vi "Timer.vi"() -> ()   [LabVIEW 2021]
uses:
  <vilib>/MakerHub/LINX/Public/Peripherals/Digital/Digital Read 1 Chan.vi
  <vilib>/MakerHub/LINX/Public/Peripherals/Digital/Digital Read N Chans.vi
  <vilib>/MakerHub/LINX/Public/Peripherals/Digital/Digital Write N Chans.vi
  <vilib>/MakerHub/LINX/Private/Local IO/LinxDigitalRead.vi
  <vilib>/MakerHub/LINX/Public/Utilities/Check Channel.vi
  <vilib>/MakerHub/LINX/Private/Local IO/LinxDigitalWrite.vi
  <vilib>/MakerHub/LINX/Public/Utilities/Open Serial.vi
  <vilib>/MakerHub/LINX/Private/Utilties/Generate Error.vi
  <vilib>/MakerHub/LINX/Public/Peripherals/Digital/Digital Write 1 Chan.vi
  <vilib>/MakerHub/LINX/LMH-LINX.lvlib
panel:
  in  "Physical Alarm Channel":u8
  out "Clock Pulse":bool
  in  "Clock Probe Channel":u8
  in  "Serial Port":refnum<visa-resource-name>="N/A"
  out "Alarm":bool
  in  "?":bool
  in  "Seconds":dbl
  in  "Minutes":dbl
  out "timer output\ntimer output":string
  in  "?":bool
  # "LINX Settings"
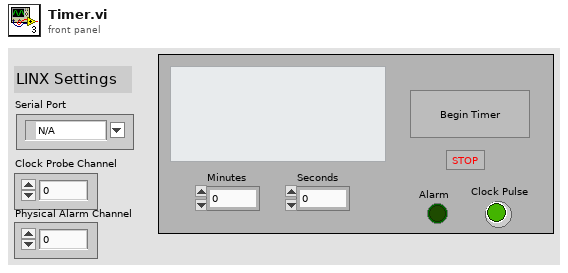
[diagram p1: front panel]
types:
  T1 = enum16{"Set Timer", "Show Running Timer", "Timer Complete", "Done"}
  T2 = typedef "LMH-LINX.lvlib/LINX Ref.ctl" = cluster{"IO":T3, "Interface":T4, "LINX Device Config":T5}
  T3 = typedef "LMH-LINX.lvlib/Platform.ctl" = enum16{"Remote", "Local"}
  T4 = typedef "LMH-LINX.lvlib/Interface.ctl" = enum16{"Serial", "TCP"}
  T5 = typedef "LMH-LINX.lvlib/Device.lvlib/LINX Device Config.ctl" = cluster{"Interface":T4, "COM Port":refnum<visa-resource-name>, "TCP Configuration":T6, "Device Family":u8, "Device ID":u8, "Device Name":string, "TCP Ref":refnum<k5>, "Channels":T7}
  T6 = typedef "LMH-LINX.lvlib/Device.lvlib/TCP Config.ctl" = cluster{"IP Address":string, "Port":u16}
  T7 = typedef "LMH-LINX.lvlib/Channels.ctl" = cluster{"DI":u8[], "DO":u8[], "AI":u8[], "AO":u8[], "PWM":u8[], "QE":u8[], "UART":u8[], "I2C 2":u8[], "SPI":u8[], "CAN":u8[], "Servo":u8[], "AI Ref (V)":dbl, "AI Resolution (Bits)":u8, "AO Ref (V)":dbl, "AO Resolution (Bits)":u8}
  T8 = enum16{"Set Timer", "Show Running Timer", "Timer Complete"}
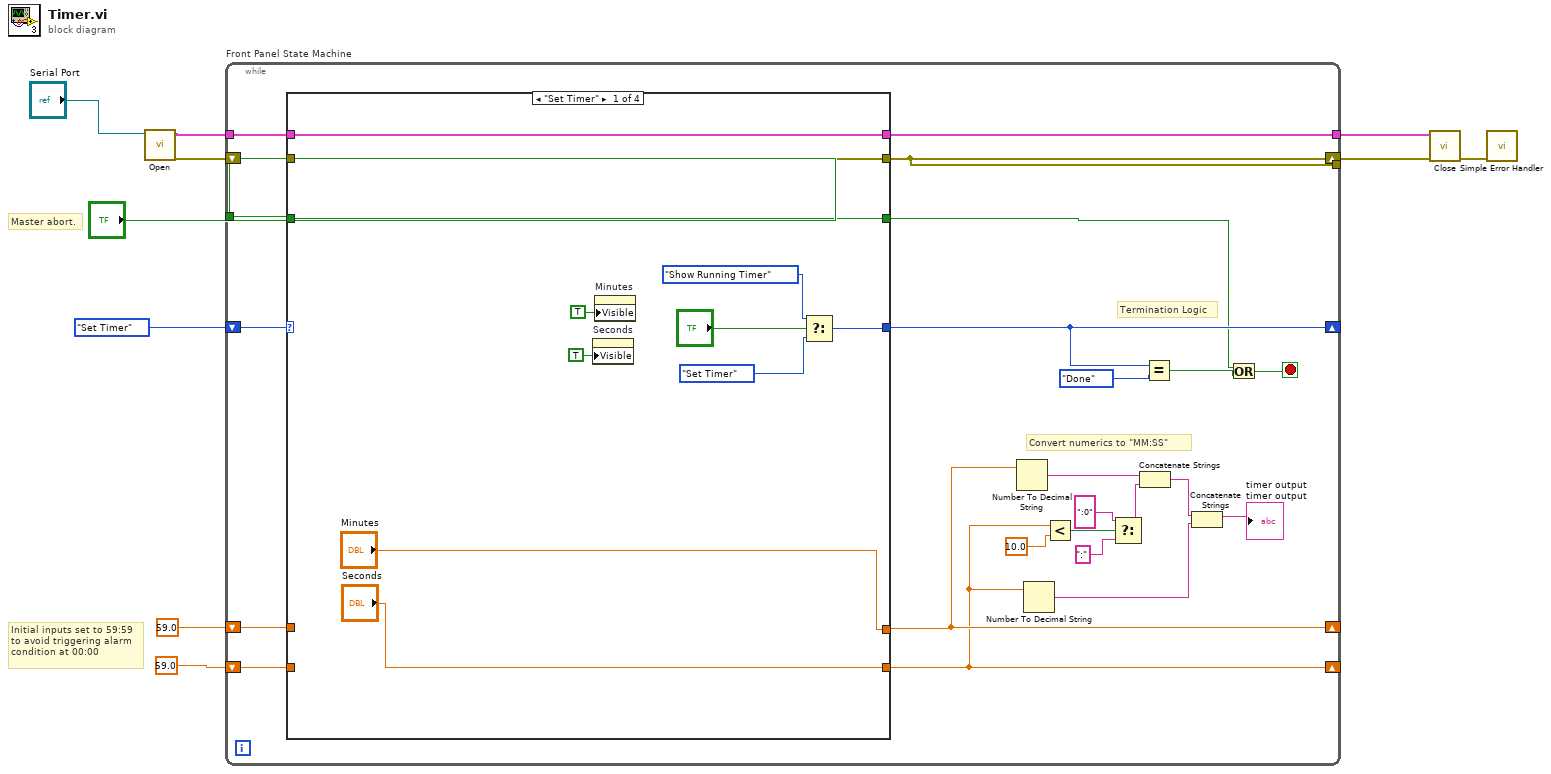
[diagram p0: block diagram]
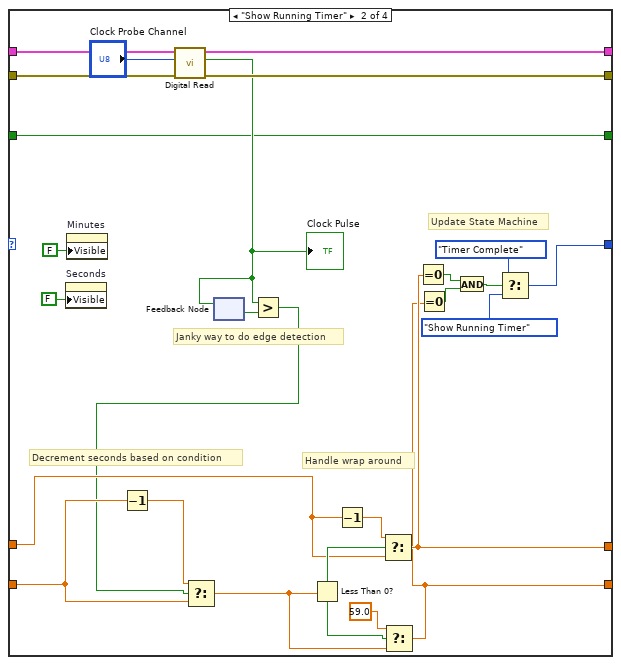
[diagram p2: hidden frame]
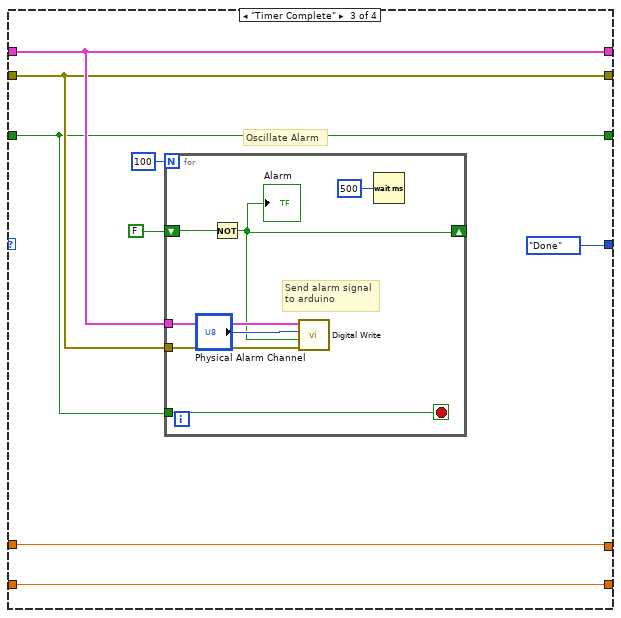
[diagram p3: hidden frame]
diagram:
  # "Initial inputs set to 59:59\nto avoid triggering alarm\ncondition at 00:00"
  # "Master abort."
  n1 = call-poly <vilib>:"Open.vi"("Serial Port"="Serial Port") -> ("Error Out"=w5:errorcluster, "LINX Resource"=w6:T2)  [unwired: 8 in, 1 out]
  n2 = while "Front Panel State Machine" {
    shift-right: [w19] -> _
    shift-left: T1."Set Timer" ("t") -> [w34]
    shift-right: [w22] -> _
    shift-left: 59.0 -> [w30]
    shift-right: [w21] -> _
    shift-left: 59.0 -> [w29]
    tunnel: "?" -> [w12]
    tunnel: w6 -> [w16]
    shift-right: [w14] -> _
    shift-left: w5 -> [w15]
    tunnel: [w14] -> w4
    tunnel: [w13] -> w3
    stop <- w17 stop-if-true
    # "Termination Logic"
    # "Convert numerics to \"MM:SS\""
    n3 = case shown="\"Set Timer\"" w34 {
      selector: w34 -> [_ _ _ w90]
      tunnel: [w43 w59 T1."Done" ("t") w90] -> w19
      tunnel: ["Minutes" w57 w75 w92] -> w22
      tunnel: ["Seconds" w56 w76 w91] -> w21
      tunnel: w30 -> [_ w66 w75 w92]
      tunnel: w29 -> [_ w55 w76 w91]
      tunnel: w12 -> [w35 w46 w72 w87]
      tunnel: w16 -> [w39 w54 w74 w89]
      tunnel: w15 -> [w38 w53 w73 w88]
      tunnel: [w38 w52 w73 w88] -> w14
      tunnel: [w39 w51 w74 w89] -> w13
      tunnel: [w35 w46 w72 w87] -> w11
      frame "Set Timer" {
        n4 = property on="Seconds" class="DigNum (strict)"("Visible"=TRUE) -> ()  [unwired: 2 in, 2 out]
        n5 = property on="Minutes" class="DigNum (strict)"("Visible"=TRUE) -> ()  [unwired: 2 in, 2 out]
        n6 = Select(t=enum16{"Set Timer", "Show Running Timer"}."Show Running Timer", s="?", f=enum16{"Set Timer", "Show Running Timer"}."Set Timer") -> (s? t:f=w43:enum16{"Set Timer", "Show Running Timer"})
      }
      frame "Show Running Timer" {
        # "Update State Machine"
        # "Janky way to do edge detection"
        # "Decrement seconds based on condition"
        # "Handle wrap around"
        n7 = property on="Seconds" class="DigNum (strict)"("Visible"=FALSE) -> ()  [unwired: 2 in, 2 out]
        n8 = property on="Minutes" class="DigNum (strict)"("Visible"=FALSE) -> ()  [unwired: 2 in, 2 out]
        n9 = Decrement(x=w55) -> (x-1=w71:dbl)
        n10 = call-poly <vilib>:"Digital Read.vi"("Error In"=w53, "DI Channel"="Clock Probe Channel", "LINX Resource"=w54) -> ("Error Out"=w52:errorcluster, "DI Value"=w47:bool, "LINX Resource"=w51:T2)  [unwired: 6 in]
        "Clock Pulse" <- w47
        n11 = feedback-in #1(w47) -> ()
        n12 = feedback #1() -> (w48:bool)  [unwired: 1 in]
        n13 = Greater?(x=w47, y=w48) -> (0:w49:bool)
        n14 = Select(t=w71, s=w49, f=w55) -> (s? t:f=w65:dbl)
        n15 = Less Than 0?(x=w65) -> (x < 0?=w68:bool)
        n16 = Decrement(x=w66) -> (x-1=w67:dbl)
        n17 = Select(t=w67, s=w68, f=w66) -> (s? t:f=w57:dbl)
        n18 = Select(t=59.0, s=w68, f=w65) -> (s? t:f=w56:dbl)
        n19 = Equal To 0?(x=w57) -> (x = 0?=w62:bool)
        n20 = Equal To 0?(x=w56) -> (x = 0?=w63:bool)
        n21 = And(x=w62, y=w63) -> (x .and. y?=w61:bool)
        n22 = Select(t=T8."Timer Complete", s=w61, f=enum16{"Set Timer", "Show Running Timer"}."Show Running Timer") -> (s? t:f=w59:T8)
      }
      frame "Timer Complete" {
        # "Oscillate Alarm"
        n23 = for {
          N: 100 -> [_]
          shift-right: [w80] -> _
          shift-left: FALSE -> [w86]
          tunnel: w72 -> [w84]
          tunnel: w74 -> [w82]
          tunnel: w73 -> [w81]
          stop <- w84 stop-if-true
          # "Send alarm signal\nto arduino"
          n24 = Not(x=w86) -> (.not. x?=w80:bool)
          "Alarm" <- w80
          n25 = call-poly <vilib>:"Digital Write.vi"("Error In"=w81, "Output Value"=w80, "DO Channel"="Physical Alarm Channel", "LINX Resource"=w82) -> ()  [unwired: 6 in, 2 out]
          n26 = Wait (ms)(milliseconds to wait=u32 500) -> ()  [unwired: 1 out]
        }
      }
      frame "Done" {
      }
    }
    n27 = Number To Decimal String(number=w22) -> (decimal integer string=w32:string)  [unwired: 1 in]
    n28 = Number To Decimal String(number=w21) -> (decimal integer string=w23:string)  [unwired: 1 in]
    n29 = Less?(x=w21, y=10.0) -> (x < y?=w25:bool)
    n30 = Select(t=":0" ("string"), s=w25, f=":" ("string")) -> (s? t:f=w27:string)
    n31 = Concatenate Strings(w32, w27) -> (w33:string)
    n32 = Equal?(x=w19, y=T1."Done" ("t")) -> (x = y?=w18:bool)
    n33 = Concatenate Strings(w33, w23) -> (→"timer output\ntimer output":string)
    n34 = Or(x=w11, y=w18) -> (x .or. y?=w17:bool)
  }
  n35 = call <vilib>:"Close.vi"("Error In"=w4, "LINX Resource"=w3) -> ("Error Out"=w2:errorcluster)  [unwired: 9 in]
  n36 = call <vilib>:"Simple Error Handler.vi"("error in (no error)"=w2) -> ()  [unwired: 4 in, 5 out]
